vi "Configure Source.vi"(0 "VISA resource name":refnum<visa-resource-name>, 1 "Channel (0: Channel 1)":i32(ring) items=["Channel 1", "Channel 2"], 3 "Source Range (2)":dbl=2.0, 5 "error in (no error)":errorcluster, 6 "Source Shape (1: DC)":i32(ring)=1 items=["Pulse", "DC"], 7 "Source Mode (1: Voltage)":i32(ring)=1 items=["Current", "Voltage"], 8 "Output Level (0)":dbl, 9 "Triggered Output Level (0)":dbl, 10 "Source Auto Range (T: Enable)":bool=TRUE, 11 "Source Range Lower Limit (2 V)":dbl=2.0, 12 "Enable Continuous Output (T: Enable)":bool=TRUE) -> (14 "VISA resource name out":refnum<visa-resource-name>, 19 "error out":errorcluster)   [LabVIEW 2020, in "Agilent B2900 Series.lvlib"]
doc: "Configures output source which includes output level, source mode, source shape, source range and enables or disables the continuous trigger sourcing."
uses:
  Agilent B2900 Series.lvlib
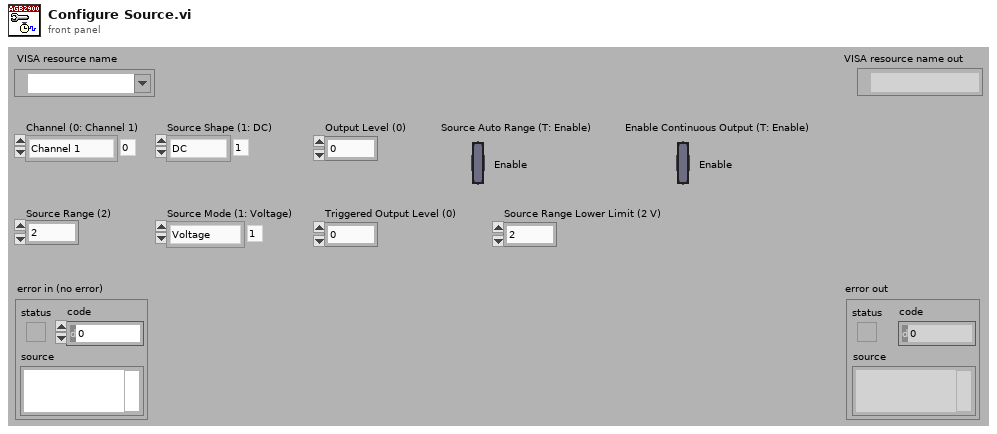
[diagram p1: front panel]
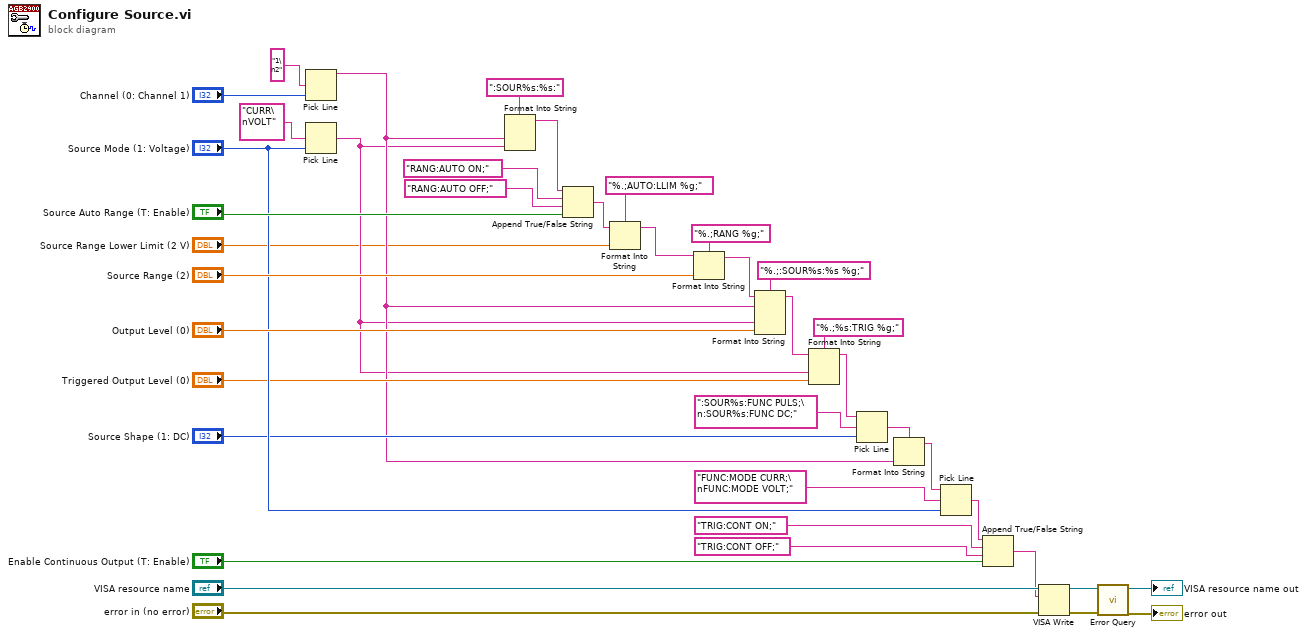
[diagram p0: block diagram]
diagram:
  n1 = Pick Line(multi-line string="1\n2" ("string (\"\")"), line index="Channel (0: Channel 1)") -> (output string=w8:string)  [unwired: 1 in]
  n2 = Pick Line(multi-line string="CURR\nVOLT" ("string (\"\")"), line index="Source Mode (1: Voltage)") -> (output string=w7:string)  [unwired: 1 in]
  n3 = Format Into String(format string=":SOUR%s:%s:", w8, w7) -> (resulting string=w5:string)  [unwired: 2 in, 1 out]
  n4 = Append True/False String(1:"Source Auto Range (T: Enable)", 2:"RANG:AUTO OFF;", 3:"RANG:AUTO ON;", 4:w5) -> (0:w2:string)
  n5 = Format Into String(format string="%.;AUTO:LLIM %g;", initial string=w2, "Source Range Lower Limit (2 V)") -> (resulting string=w4:string)  [unwired: 1 in, 1 out]
  n6 = Format Into String(format string="%.;RANG %g;", initial string=w4, "Source Range (2)") -> (resulting string=w15:string)  [unwired: 1 in, 1 out]
  n7 = Format Into String(format string="%.;:SOUR%s:%s %g;", initial string=w15, w8, w7, "Output Level (0)") -> (resulting string=w38:string)  [unwired: 1 in, 1 out]
  n8 = Format Into String(format string="%.;%s:TRIG %g;", initial string=w38, w7, "Triggered Output Level (0)") -> (resulting string=w14:string)  [unwired: 1 in, 1 out]
  n9 = Pick Line(string ("")=w14, multi-line string=":SOUR%s:FUNC PULS;\n:SOUR%s:FUNC DC;", line index="Source Shape (1: DC)") -> (output string=w22:string)
  n10 = Format Into String(format string=w22, w8) -> (resulting string=w21:string)  [unwired: 2 in, 1 out]
  n11 = Pick Line(string ("")=w21, multi-line string="FUNC:MODE CURR;\nFUNC:MODE VOLT;", line index="Source Mode (1: Voltage)") -> (output string=w20:string)
  n12 = Append True/False String(1:"Enable Continuous Output (T: Enable)", 2:"TRIG:CONT OFF;", 3:"TRIG:CONT ON;", 4:w20) -> (0:w10:string)
  n13 = VISA Write(VISA resource name="VISA resource name", write buffer=w10, error in (no error)="error in (no error)") -> (VISA resource name out=w29:refnum<visa-resource-name>, error out=w28:errorcluster)  [unwired: 1 out]
  n14 = call "Error Query.vi"("error in (no error)"=w28, "VISA resource name"=w29) -> ("error out"=→"error out":errorcluster, "VISA resource name out"=→"VISA resource name out":refnum<visa-resource-name>)  [unwired: 6 in, 2 out]
